vi "生成2和4.vi"(10 "索引数组":cluster{"行":i32, "列":i32}[](array[cluster]), 11 "2048输入":i32[][](array[numeric])) -> (3 "2048输出":i32[][](array[numeric]))   [LabVIEW 2020]
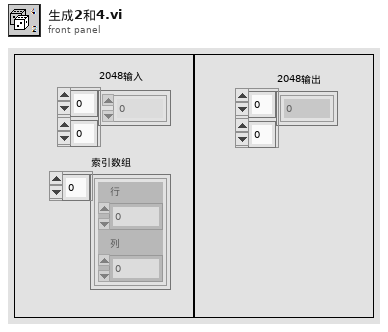
[diagram p1: front panel]
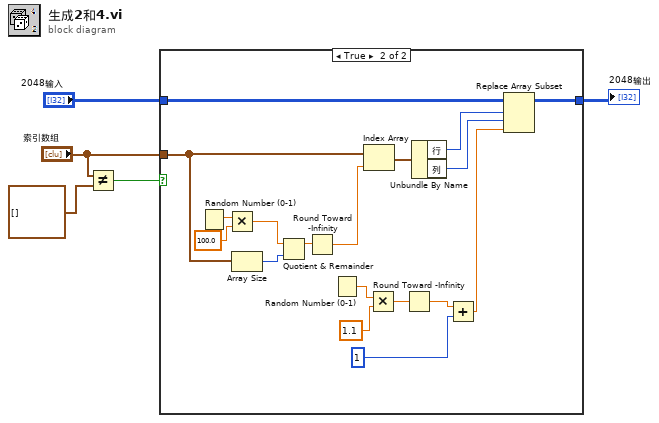
[diagram p0: block diagram]
diagram:
  n1 = Not Equal?(x="索引数组", y=cluster{"行":i32, "列":i32}[] []) -> (x != y?=w1:bool)
  n2 = case shown="True" w1 {
    tunnel: "2048输入" -> [w6 w18]
    tunnel: [w6 w14] -> w4
    tunnel: "索引数组" -> [_ w13]
    frame False {
    }
    frame True {
      n3 = Random Number (0-1)() -> (number: 0 to 1=w24:dbl)
      n4 = Multiply(x=w24, y=100.0) -> (x*y=w21:dbl)
      n5 = Array Size(array=w13) -> (size(s)=w22:i32)
      n6 = Quotient & Remainder(x=w21, y=w22) -> (x-y*floor(x/y)=w20:dbl)  [unwired: 1 out]
      n7 = Round Toward -Infinity(1:w20) -> (0:w19:dbl)
      n8 = Random Number (0-1)() -> (number: 0 to 1=w11:dbl)
      n9 = Index Array(array=w13, index=w19) -> (element=w17:cluster{"行":i32, "列":i32})
      n10 = Multiply(x=w11, y=1.1) -> (x*y=w10:dbl)
      n11 = Round Toward -Infinity(1:w10) -> (0:w8:dbl)
      n12 = Unbundle By Name(w17) -> ("行"=w16:i32, "列"=w15:i32)
      n13 = Add(x=w8, y=1) -> (x+y=w7:dbl)
      n14 = Replace Array Subset(array=w18, new element=w7, index (row)=w16, index (col)=w15) -> (w14:i32[][])
    }
  }
  "2048输出" <- w4
